vi "Globals.vi"() -> ()   [LabVIEW 2012, in "TIFF File Reader.lvlib"]
uses:
  TIFF File Reader.lvlib
panel:
  in  "Litt/BigEnd":bool
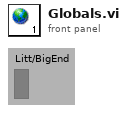
[diagram p1: front panel]
diagram:
